vi "20TVTIMonitor.vi"() -> ()   [LabVIEW 2019]
uses:
  Utility/Monitor Communication/Gustav/20TVTI_Cluster.ctl
  Utility/Monitor Communication/Gustav/20TVTI_Control.ctl
  Instrument_Setup.vi
  Global/Global Variables/Data_Display_global.vi
  Equipment/Mercury iXX/Public/Libraries/Heater/Open/Open Heater Device.vi
  Equipment/Mercury iXX/Public/Libraries/Heater/Signals/Read/Voltage (Read).vi
  Equipment/Mercury iXX/Public/Libraries/Temperature/Open/Open Temperature Device.vi
  Equipment/Mercury iXX/Public/Libraries/Temperature/Signals/Read/Temperature (Read).vi
  Equipment/Mercury iXX/Public/Libraries/Auxiliary/Open/Open Auxiliary Device.vi
  Equipment/Mercury iXX/Public/Libraries/Auxiliary/Signals/Read/Percent Open (Read).vi
  Equipment/Mercury iXX/Public/Libraries/Temperature/Signals/Read/Status (Read).vi
  Equipment/Mercury iXX/Public/Libraries/Temperature/Signals/Read/Status Heater (Read).vi
  Utility/Monitor Communication/sub-vis/20TVTI-Set-T.vi
  Utility/Monitor Communication/sub-vis/20TVTI-Change_Sweep_Mode.vi
  Utility/Monitor Communication/sub-vis/20TVTI-Set-Htr-VTI.vi
  Utility/Monitor Communication/sub-vis/20TVTI-Set-Heater-Manual.vi
  Utility/Monitor Communication/sub-vis/20TVTI-Set-NV-Value.vi
  Utility/Monitor Communication/sub-vis/20TVTI-Set-NV-Manual.vi
  Equipment/Mercury iXX/Mercury iXX.lvlib
  Equipment/Mercury iXX/Public/Libraries/Heater.lvlib
  Equipment/Mercury iXX/Public/Libraries/Temperature.lvlib
  Equipment/Mercury iXX/Public/Libraries/Auxiliary.lvlib
  Equipment/Mercury iXX/Public/Libraries/Control Loop.lvlib
panel:
  out "20TVTI":T1={"Temperatur (K)"=0.0, "Setpoint (K)"=0.0, "Rate (K/min)"=3.4572, "Heater (%)"=0.0, "NV (%)"=0.0, "Heater Manual"=FALSE, "NV Manual"=FALSE, "Go to Set"=FALSE, "Heater SP"=0.0, "Valid?"=FALSE, "Set Heater SP"=FALSE, "Set NV SP"=FALSE, "Heater (%) Display"=3.4572, "NV (%) Display"=3.4572, "NV Setpoint"=0.0, "Change Heater Status"=FALSE, "Change NV Status"=FALSE, "Stop"=FALSE, "Current T Setpoint"=0.0, "Sweeping?"=FALSE, "Ramp Mode"="", "Change Sweep Mode"=FALSE} {"Current T Setpoint" format="%#.3g"; "NV (%) Display" format="%4.1f"; "Heater (%) Display" format="%4.1f"; "NV (%)" scale=0.0..100.0; "Heater (%)" scale=0.0..100.0; "Rate (K/min)" format="%#4_5f"; "Setpoint (K)" format="%6.3f"; "Temperatur (K)" format="%.3g"}
  in  "local error":errorcluster
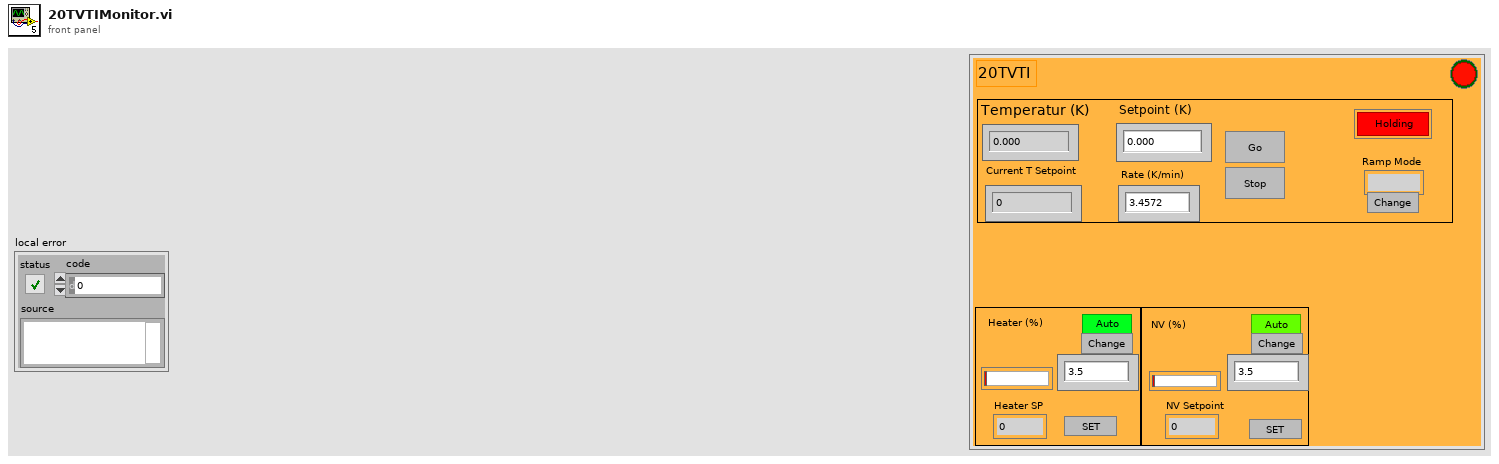
[diagram p1: front panel]
types:
  T1 = typedef "20TVTI_Cluster.ctl" = cluster{"Temperatur (K)":dbl, "Setpoint (K)":dbl, "Rate (K/min)":dbl, "Heater (%)":dbl, "NV (%)":dbl, "Heater Manual":bool, "NV Manual":bool, "Go to Set":bool, "Heater SP":dbl, "Valid?":bool, "Set Heater SP":bool, "Set NV SP":bool, "Heater (%) Display":dbl, "NV (%) Display":dbl, "NV Setpoint":dbl, "Change Heater Status":bool, "Change NV Status":bool, "Stop":bool, "Current T Setpoint":dbl, "Sweeping?":bool, "Ramp Mode":string, "Change Sweep Mode":bool}
  T2 = typedef "20TVTI_Control.ctl" = cluster{"Set VTI SP":bool, "Change NV Status":bool, "Set NV Setpoint":bool, "Change Heater Status":bool, "Set Heater Setpoint":bool, "Stop Sweep":bool, "Setpoint (K)":dbl, "Rate (K/min)":dbl, "Setpoint Heater":dbl, "Setpoint NV":dbl, "Change Sweep Mode":bool}
  T3 = typedef "Mercury iXX.lvlib/Mercury Reference.ctl" = cluster{"Comms":refnum<visa-resource-name>, "Device ID":string[], "Comms Layer":T4, "Command":string, "Query reference":T5}
  T4 = typedef "Mercury iXX.lvlib/Comms Transport Layer.ctl" = enum16{"Ethernet TCP/IP", "USB", "ISOBus - RS-232", "GPIB"}
  T5 = typedef "Mercury iXX.lvlib/Query Dynamic Reference.ctl" = refnum<vi>
  T6 = typedef "Mercury iXX.lvlib/Unit String.ctl" = string
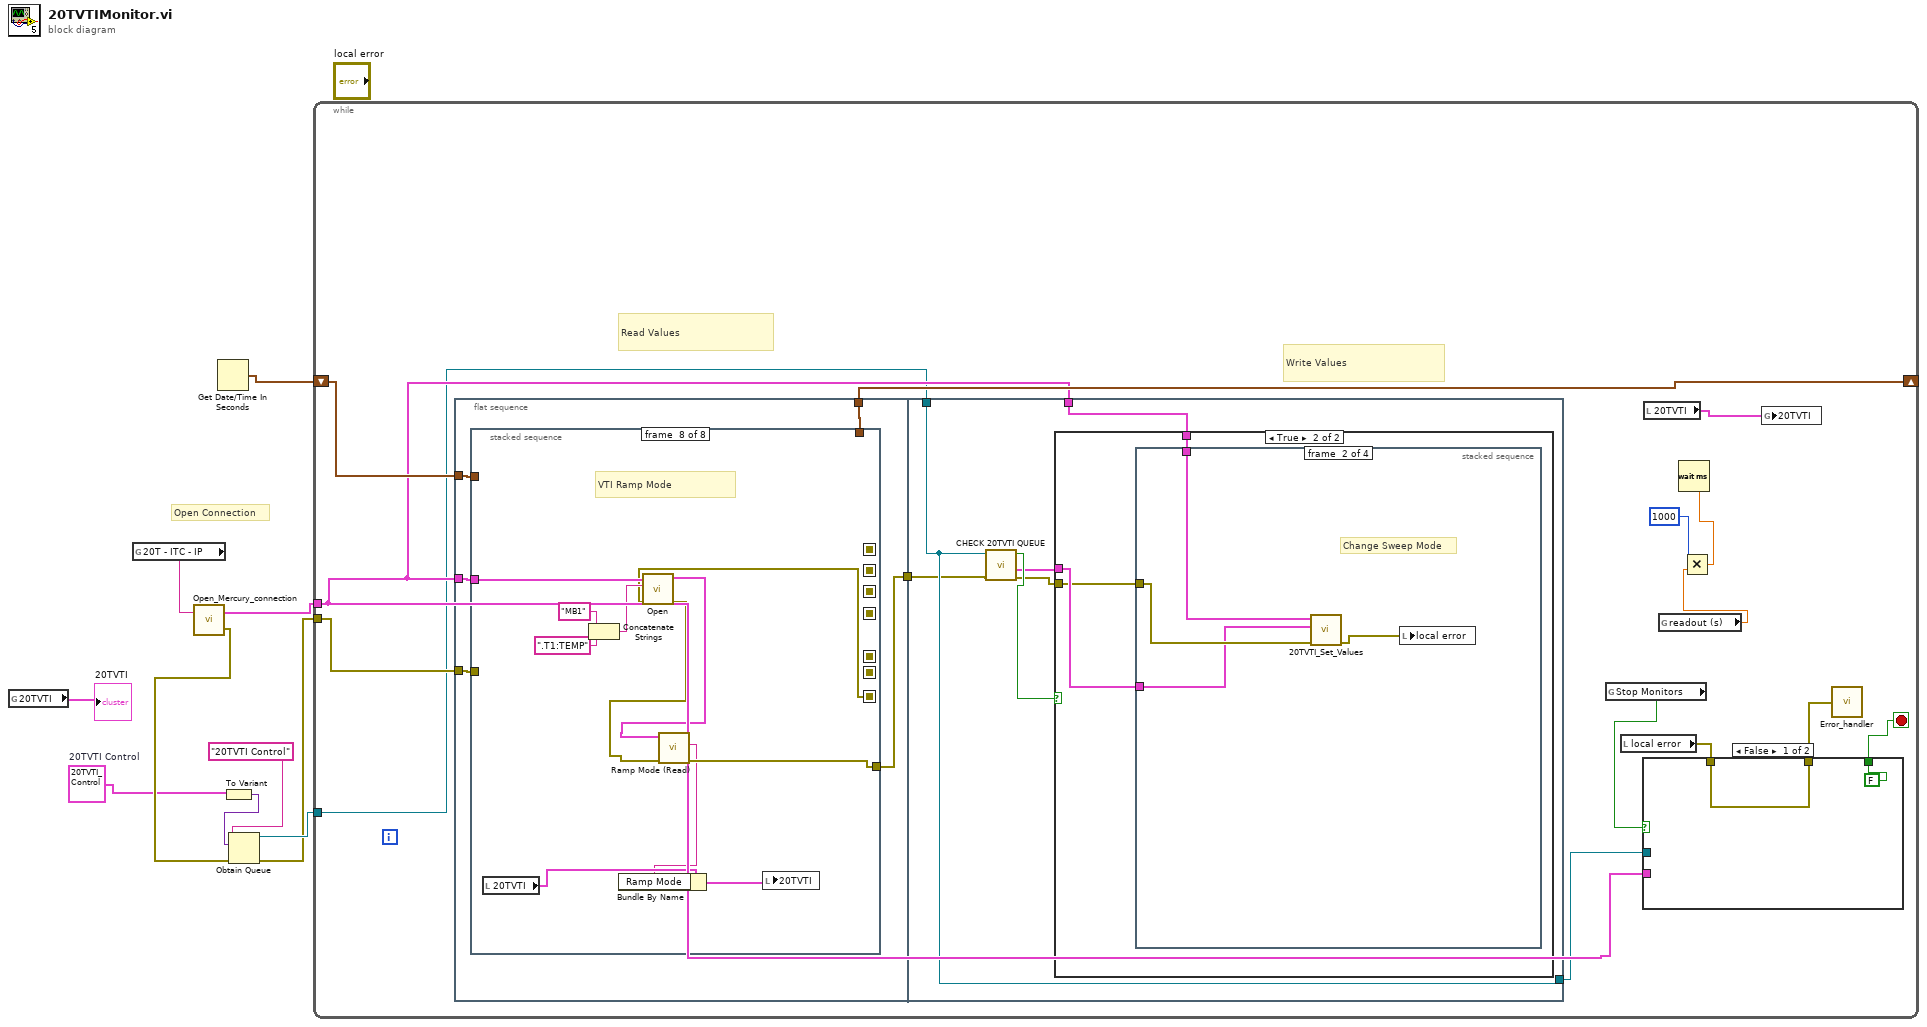
[diagram p0: block diagram]
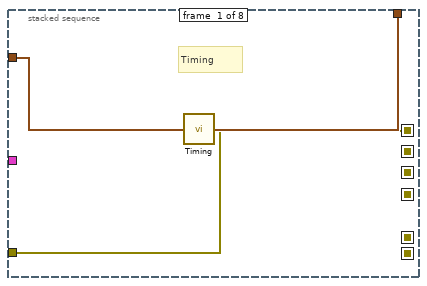
[diagram p2: hidden frame]
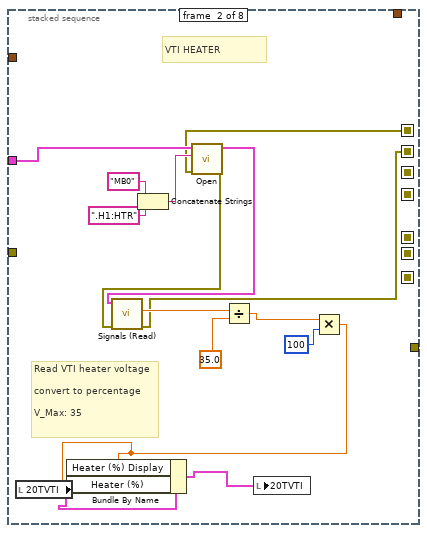
[diagram p3: hidden frame]
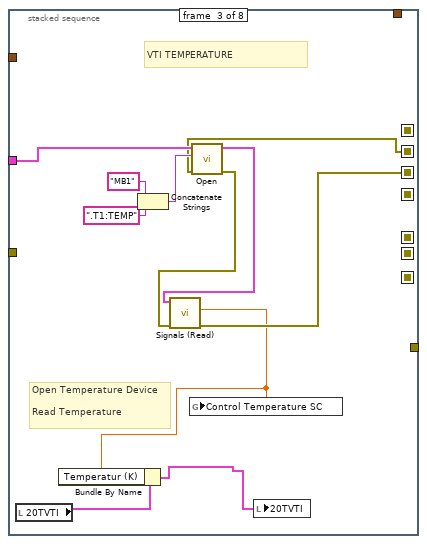
[diagram p4: hidden frame]
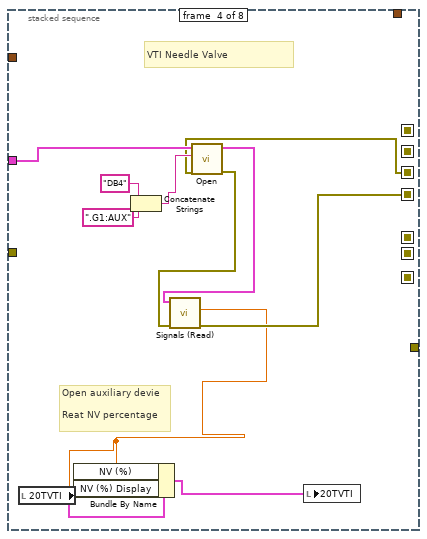
[diagram p5: hidden frame]
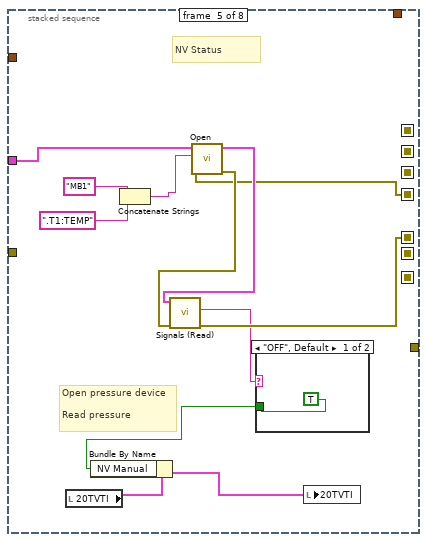
[diagram p6: hidden frame]
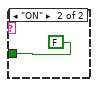
[diagram p7: hidden frame]
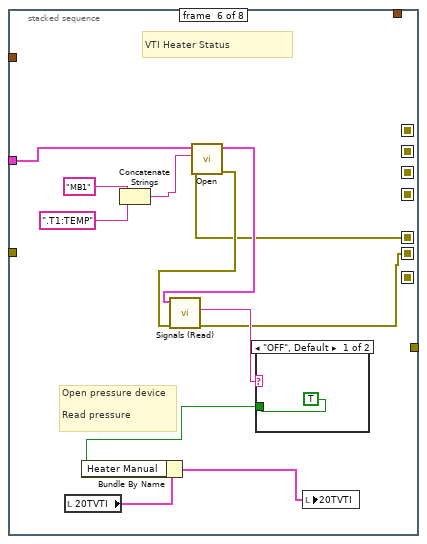
[diagram p8: hidden frame]
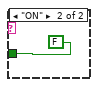
[diagram p9: hidden frame]
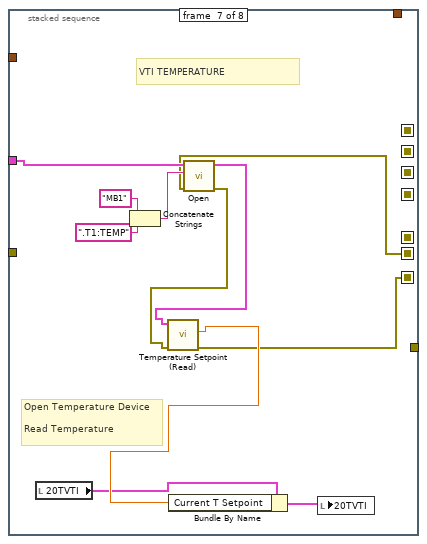
[diagram p10: hidden frame]
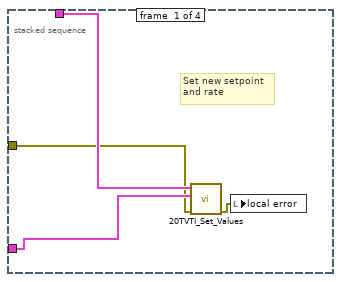
[diagram p12: hidden frame]
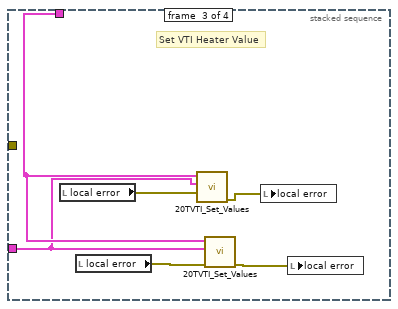
[diagram p13: hidden frame]
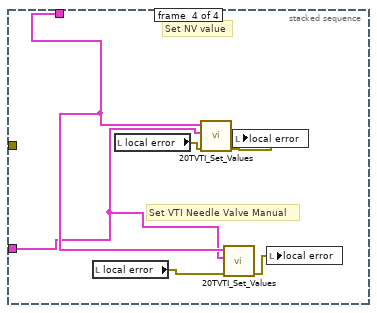
[diagram p14: hidden frame]
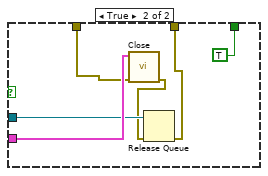
[diagram p15: hidden frame]
diagram:
  w1 = T2 {"Set VTI SP"=FALSE, "Change NV Status"=FALSE, "Set NV Setpoint"=FALSE, "Change Heater Status"=FALSE, "Set Heater Setpoint"=FALSE, "Stop Sweep"=FALSE, "Setpoint (K)"=0.0, "Rate (K/min)"=0.0, "Setpoint Heater"=0.0, "Setpoint NV"=0.0, "Change Sweep Mode"=FALSE}  # 20TVTI Control
  # "Open Connection"
  n1 = global read "Data_Display_global.vi" "20TVTI"() -> (→"20TVTI":T1)
  n2 = global read "Instrument_Setup.vi" "20T - ITC - IP"() -> (w9:string)
  n3 = call "Open_Mercury_connection.vi"("IP Address"=w9) -> ("error out"=w3:errorcluster, "Mercury Reference Out"=w10:T3)  [unwired: 1 in]
  n4 = Get Date/Time In Seconds() -> (seconds since 1Jan1904=w8:timestamp)
  n5 = To Variant(anything=w1) -> (Variant=w7:variant)
  n6 = Obtain Queue(name (unnamed)="20TVTI Control", element data type=w7, error in (no error)=w3) -> (queue out=w5:refnum<queue>, error out=w2:errorcluster)  [unwired: 2 in, 1 out]
  n7 = while {
    tunnel: w10 -> [w15]
    tunnel: w2 -> [w25]
    shift-right: [w17] -> _
    shift-left: w8 -> [w18]
    tunnel: w5 -> [w13]
    stop <- w21 stop-if-true
    # "Write Values"
    # "Read Values"
    n8 = flat-sequence {
      tunnel: w25 -> [w30]
      tunnel: w15 -> [w29]
      tunnel: w18 -> [w28]
      tunnel: [w27] -> w17
      tunnel: [w26] -> w11
      tunnel: w15 -> [w126]
      tunnel: w13 -> [w125]
      tunnel: [w125] -> w12
      tunnel: w11 -> [w124]
      frame #0 {
        n9 = stacked-sequence {
          seq-local: [w31 _ _ _ _ _ _ _] -> [_ w38 _ _ _ _ _ _]
          seq-local: [_ w37 _ _ _ _ _ _] -> [_ _ w53 _ _ _ _ _]
          seq-local: [_ _ w52 _ _ _ _ _] -> [_ _ _ w64 _ _ _ _]
          seq-local: [_ _ _ w63 _ _ _ _] -> [_ _ _ _ w71 _ _ _]
          seq-local: [_ _ _ _ w75 _ _ _] -> [_ _ _ _ _ w88 _ _]
          seq-local: [_ _ _ _ _ w85 _ _] -> [_ _ _ _ _ _ w100 _]
          seq-local: [_ _ _ _ _ _ w99 _] -> [_ _ _ _ _ _ _ w114]
          tunnel: w29 -> [_ w46 w57 w70 w82 w96 w101 w117]
          tunnel: w30 -> [w31 _ _ _ _ _ _ _]
          tunnel: w28 -> [w33 _ _ _ _ _ _ _]
          tunnel: [w32 _ _ _ _ _ _ _] -> w27
          tunnel: [_ _ _ _ _ _ _ w111] -> w26
          frame #0 {
            # "Timing"
            n10 = call "Timing.vi"("start time (s)"=w33) -> ("last reading (s)"=w32:timestamp)
          }
          frame #1 {
            # "VTI HEATER"
            # "Read VTI heater voltage\n\nconvert to percentage\n\nV_Max: 35"
            n11 = local read "20TVTI"() -> (w35:T1)
            n12 = Concatenate Strings("MB0", ".H1:HTR" ("Device Identifier")) -> (w45:string)
            n13 = call-poly "Open.vi"("error in (no error)"=w38, "Device Identifier"=w45, "Mercury Reference In"=w46) -> ("error out"=w39:errorcluster, "Mercury Reference Out"=w40:T3)  [unwired: 1 in, 6 out]
            n14 = call-poly "Signals (Read).vi"("error in"=w39, "Mercury Reference In"=w40) -> ("error out"=w37:errorcluster, "Voltage"=w41:dbl)  [unwired: 5 in, 3 out]
            n15 = Divide(x=w41, y=35.0) -> (x/y=w43:dbl)
            n16 = Multiply(x=w43, y=100) -> (x*y=w36:dbl)
            n17 = Bundle By Name(cluster=w35, "Heater (%) Display"=w36, "Heater (%)"=w36) -> (w34:T1)
            n18 = local write "20TVTI"(w34) -> ()
          }
          frame #2 {
            # "Open Temperature Device\n\nRead Temperature"
            # "VTI TEMPERATURE"
            n19 = local read "20TVTI"() -> (w50:T1)
            n20 = Concatenate Strings("MB1", ".T1:TEMP" ("Device Identifier")) -> (w56:string)
            n21 = call-poly "Open.vi"("error in (no error)"=w53, "Device Identifier"=w56, "Mercury Reference In"=w57) -> ("error out"=w54:errorcluster, "Mercury Reference Out"=w55:T3)  [unwired: 1 in, 6 out]
            n22 = call-poly "Signals (Read).vi"("error in"=w54, "Mercury Reference In"=w55) -> ("error out"=w52:errorcluster, "Temperature"=w51:dbl)  [unwired: 5 in, 3 out]
            n23 = Bundle By Name(cluster=w50, "Temperatur (K)"=w51) -> (w49:T1)
            n24 = global write "Data_Display_global.vi" "Control Temperature SC"(w51) -> ()
            n25 = local write "20TVTI"(w49) -> ()
          }
          frame #3 {
            # "Open auxiliary devie\n\nReat NV percentage"
            # "VTI Needle Valve"
            n26 = local read "20TVTI"() -> (w61:T1)
            n27 = Concatenate Strings("DB4", ".G1:AUX" ("Device Identifier")) -> (w65:string)
            n28 = call-poly "Open.vi"("error in (no error)"=w64, "Device Identifier"=w65, "Mercury Reference In"=w70) -> ("error out"=w68:errorcluster, "Mercury Reference Out"=w69:T3)  [unwired: 1 in, 6 out]
            n29 = call-poly "Signals (Read).vi"("error in"=w68, "Mercury Reference In"=w69) -> ("error out"=w63:errorcluster, "% Open"=w62:dbl)  [unwired: 5 in, 3 out]
            n30 = Bundle By Name(cluster=w61, "NV (%)"=w62, "NV (%) Display"=w62) -> (w60:T1)
            n31 = local write "20TVTI"(w60) -> ()
          }
          frame #4 {
            # "Open pressure device\n\nRead pressure"
            # "NV Status"
            n32 = local read "20TVTI"() -> (w73:T1)
            n33 = Concatenate Strings("MB1", ".T1:TEMP" ("Device Identifier")) -> (w77:string)
            n34 = call-poly "Open.vi"("error in (no error)"=w71, "Device Identifier"=w77, "Mercury Reference In"=w82) -> ("error out"=w80:errorcluster, "Mercury Reference Out"=w81:T3)  [unwired: 1 in, 6 out]
            n35 = call-poly "Signals (Read).vi"("error in"=w80, "Mercury Reference In"=w81) -> ("error out"=w75:errorcluster, "State"=w74:T6)  [unwired: 6 in, 2 out]
            n36 = case shown="\"OFF\", Default" w74 {
              tunnel: [TRUE FALSE] -> w76
              frame "OFF", Default {
              }
              frame "ON" {
              }
            }
            n37 = Bundle By Name(cluster=w73, "NV Manual"=w76) -> (w72:T1)
            n38 = local write "20TVTI"(w72) -> ()
          }
          frame #5 {
            # "Open pressure device\n\nRead pressure"
            # "VTI Heater Status"
            n39 = local read "20TVTI"() -> (w87:T1)
            n40 = Concatenate Strings("MB1", ".T1:TEMP" ("Device Identifier")) -> (w91:string)
            n41 = call-poly "Open.vi"("error in (no error)"=w88, "Device Identifier"=w91, "Mercury Reference In"=w96) -> ("error out"=w94:errorcluster, "Mercury Reference Out"=w95:T3)  [unwired: 1 in, 6 out]
            n42 = call-poly "Signals (Read).vi"("error in"=w94, "Mercury Reference In"=w95) -> ("error out"=w85:errorcluster, "State"=w90:T6)  [unwired: 6 in, 2 out]
            n43 = case shown="\"OFF\", Default" w90 {
              tunnel: [TRUE FALSE] -> w89
              frame "OFF", Default {
              }
              frame "ON" {
              }
            }
            n44 = Bundle By Name(cluster=w87, "Heater Manual"=w89) -> (w86:T1)
            n45 = local write "20TVTI"(w86) -> ()
          }
          frame #6 {
            # "Open Temperature Device\n\nRead Temperature"
            # "VTI TEMPERATURE"
            n46 = local read "20TVTI"() -> (w103:T1)
            n47 = Concatenate Strings("MB1", ".T1:TEMP" ("Device Identifier")) -> (w107:string)
            n48 = call-poly "Open.vi"("error in (no error)"=w100, "Device Identifier"=w107, "Mercury Reference In"=w101) -> ("error out"=w105:errorcluster, "Mercury Reference Out"=w106:T3)  [unwired: 1 in, 6 out]
            n49 = call "Temperature Setpoint (Read).vi"("error in"=w105, "Mercury Reference In"=w106) -> ("error out"=w99:errorcluster, "Temperature Setpoint"=w104:dbl)  [unwired: 5 in, 3 out]
            n50 = Bundle By Name(cluster=w103, "Current T Setpoint"=w104) -> (w102:T1)
            n51 = local write "20TVTI"(w102) -> ()
          }
          frame #7 {
            # "VTI Ramp Mode"
            n52 = local read "20TVTI"() -> (w116:T1)
            n53 = Concatenate Strings("MB1", ".T1:TEMP" ("Device Identifier")) -> (w118:string)
            n54 = call-poly "Open.vi"("error in (no error)"=w114, "Device Identifier"=w118, "Mercury Reference In"=w117) -> ("error out"=w112:errorcluster, "Mercury Reference Out"=w113:T3)  [unwired: 1 in, 6 out]
            n55 = call "Ramp Mode (Read).vi"("error in"=w112, "Mercury Reference In"=w113) -> ("error out"=w111:errorcluster, "Sweep Mode"=w110:string)  [unwired: 6 in, 2 out]
            n56 = Bundle By Name(cluster=w116, "Ramp Mode"=w110) -> (w115:T1)
            n57 = local write "20TVTI"(w115) -> ()
          }
        }
      }
      frame #1 {
        n58 = call "CHECK 20TVTI QUEUE.vi"("error in (no error)"=w124, "queue"=w125) -> ("error out"=w122:errorcluster, "VTI Control"=w121:T2, "New Entries?"=w123:bool)  [unwired: 6 in]
        n59 = case shown="True" w123 {
          tunnel: w126 -> [_ w129]
          tunnel: w121 -> [_ w128]
          tunnel: w122 -> [_ w127]
          frame False {
          }
          frame True {
            n60 = stacked-sequence {
              tunnel: w129 -> [w132 w135 w139 w145]
              tunnel: w128 -> [w131 w136 w138 w144]
              tunnel: w127 -> [w130 w137 _ _]
              frame #0 {
                # "Set new setpoint \nand rate"
                n61 = call-poly "20TVTI_Set_Values.vi"("error in (no error)"=w130, "20TVTI Control"=w131, "Mercury Reference In"=w132) -> ("error out"=w133:errorcluster)  [unwired: 8 in]
                n62 = local write "local error"(w133) -> ()
              }
              frame #1 {
                # "Change Sweep Mode"
                n63 = call-poly "20TVTI_Set_Values.vi"("error in (no error)"=w137, "20TVTI Control"=w136, "Mercury Reference In"=w135) -> ("error out"=w134:errorcluster)  [unwired: 8 in]
                n64 = local write "local error"(w134) -> ()
              }
              frame #2 {
                # "Set VTI Heater Value"
                n65 = local read "local error"() -> (w143:errorcluster)
                n66 = local read "local error"() -> (w141:errorcluster)
                n67 = call-poly "20TVTI_Set_Values.vi"("error in (no error)"=w143, "20TVTI Control"=w138, "Mercury Reference In"=w139) -> ("error out"=w142:errorcluster)  [unwired: 8 in]
                n68 = call-poly "20TVTI_Set_Values.vi"("error in (no error)"=w141, "20TVTI Control"=w138, "Mercury Reference In"=w139) -> ("error out"=w140:errorcluster)  [unwired: 8 in]
                n69 = local write "local error"(w142) -> ()
                n70 = local write "local error"(w140) -> ()
              }
              frame #3 {
                # "Set VTI Needle Valve Manual"
                # "Set NV value"
                n71 = local read "local error"() -> (w147:errorcluster)
                n72 = local read "local error"() -> (w149:errorcluster)
                n73 = call-poly "20TVTI_Set_Values.vi"("error in (no error)"=w149, "20TVTI Control"=w144, "Mercury Reference In"=w145) -> ("error out"=w148:errorcluster)  [unwired: 8 in]
                n74 = call-poly "20TVTI_Set_Values.vi"("error in (no error)"=w147, "20TVTI Control"=w144, "Mercury Reference In"=w145) -> ("error out"=w146:errorcluster)  [unwired: 8 in]
                n75 = local write "local error"(w148) -> ()
                n76 = local write "local error"(w146) -> ()
              }
            }
          }
        }
      }
    }
    n77 = global read "Data_Display_global.vi" "Stop Monitors"() -> (w19:bool)
    n78 = local read "local error"() -> (w16:errorcluster)
    n79 = case shown="False" w19 {
      tunnel: w15 -> [_ w157]
      tunnel: [w150 w152] -> w20
      tunnel: [FALSE TRUE] -> w21
      tunnel: w16 -> [w150 w155]
      tunnel: w12 -> [_ w154]
      frame False {
      }
      frame True {
        n80 = call "Close.vi"("error in (no error)"=w155, "Mercury Reference"=w157) -> ("error out"=w153:errorcluster)  [unwired: 9 in]
        n81 = Release Queue(queue=w154, error in (no error)=w153) -> (error out=w152:errorcluster)  [unwired: 1 in, 2 out]
      }
    }
    n82 = local read "20TVTI"() -> (w14:T1)
    n83 = global read "Instrument_Setup.vi" "readout (s)"() -> (w24:dbl)
    n84 = Multiply(x=1000, y=w24) -> (x*y=w23:dbl)
    n85 = Wait (ms)(milliseconds to wait=w23) -> ()  [unwired: 1 out]
    n86 = global write "Data_Display_global.vi" "20TVTI"(w14) -> ()
    n87 = call "Error_handler.vi"("error constant"=w20) -> ()
  }
